vi "hamamatsu_shutdown.vi"(8 "error in (no error)":errorcluster, 10 "Use camera?":bool=TRUE, 11 "IMAQ Session In":refnum<k11>) -> (0 "error out":errorcluster)   [LabVIEW 2013]
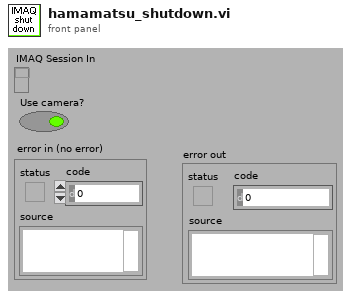
[diagram p1: front panel]
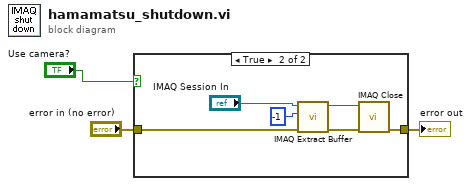
[diagram p0: block diagram]
diagram:
  n1 = case shown="True" "Use camera?" {
    tunnel: "error in (no error)" -> [w4 w8]
    tunnel: [w4 w6] -> w2
    frame False {
    }
    frame True {
      n2 = call <vilib>:"IMAQ Extract Buffer.vi"("error in (no error)"=w8, "Buffer to extract"=-1, "IMAQ Session In"="IMAQ Session In") -> ("error out"=w10:errorcluster, "IMAQ Session Out"=w9:refnum<k11>)  [unwired: 3 in, 4 out]
      n3 = call <vilib>:"IMAQ Close.vi"("error in (no error)"=w10, "IMAQ Session In"=w9) -> ("error out"=w6:errorcluster)  [unwired: 9 in]
    }
  }
  "error out" <- w2
